vi "Sgl_ErrorCodes&Descs.vi"() -> (0 "Sgl_ErrorsDescs_Trans":T1(array[cluster]) caption="Avantes Error Descriptions (Translated Codes)")   [LabVIEW 2012, in "SG-Lock.lvlib"]
uses:
  SG-Lock.lvlib
panel:
  out "Sgl_ErrorsDescs":T2(array[cluster])=[{"Code"=1, "Name"=enum."SGL_DGL_NOT_FOUND", "Description"="SG-Lock not found"}, {"Code"=2, "Name"=enum."SGL_LPT_BUSY", "Description"="At least one LPT-Port is used by another program and on the other ports no SG-Lock was found"}, {"Code"=3, "Name"=enum."SGL_LPT_OPEN_ERROR", "Description"="The SG-Lock LPT-driver was not found, even though the SGLock LPT support is installed"}, {"Code"=4, "Name"=enum."SGL_NO_LPT_PORT_FOUND", "Description"="There is no LPT-Port installed in the PC, even though the SG-Lock LPT support is installed"}, {"Code"=5, "Name"=enum."SGL_AUTHENTICATION_REQUIRED", "Description"="Authentication with SglAuthent() not or not errorfree processed"}, {"Code"=6, "Name"=enum."SGL_AUTHENTICATION_FAILED", "Description"="Authentication with SglAuthent() failed"}, {"Code"=7, "Name"=enum."SGL_FUNCTION_NOT_SUPPORTED", "Description"="The called function is not supported by the found SG-Lock"}, {"Code"=8, "Name"=enum."SGL_PARAMETER_INVALD", "Description"="Parameter of the called function is out of the vaild value range"}, {"Code"=9, "Name"=enum."SGL_SIGNATURE_INVALID", "Description"="Signature invalid"}, {"Code"=10, "Name"=enum."SGL_USB_BUSY", "Description"="Another application is claming the SG-Lock for more than 5 seconds"}] caption="Avantes Error Descriptions (Directly from Doc)"
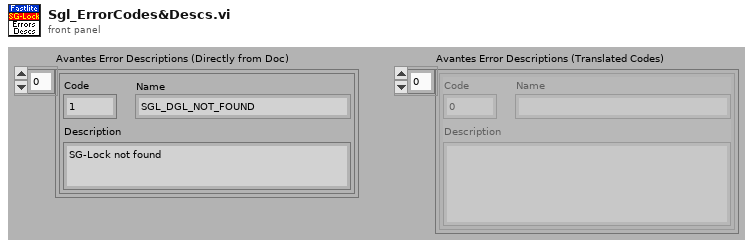
[diagram p1: front panel]
types:
  T1 = cluster{"Code":i32, "Name":string, "Description":string}[]
  T2 = cluster{"Code":i32, "Name":enum16{"SGL_SUCCESS", "SGL_DGL_NOT_FOUND", "SGL_LPT_BUSY", "SGL_LPT_OPEN_ERROR", "SGL_NO_LPT_PORT_FOUND", "SGL_AUTHENTICATION_REQUIRED", "SGL_AUTHENTICATION_FAILED", "SGL_FUNCTION_NOT_SUPPORTED", "SGL_PARAMETER_INVALD", "SGL_SIGNATURE_INVALID", "SGL_USB_BUSY"}, "Description":string}[]
  T3 = cluster{"Code":i32, "Name":string, "Description":string}
  T4 = enum16{"SGL_SUCCESS", "SGL_DGL_NOT_FOUND", "SGL_LPT_BUSY", "SGL_LPT_OPEN_ERROR", "SGL_NO_LPT_PORT_FOUND", "SGL_AUTHENTICATION_REQUIRED", "SGL_AUTHENTICATION_FAILED", "SGL_FUNCTION_NOT_SUPPORTED", "SGL_PARAMETER_INVALD", "SGL_SIGNATURE_INVALID", "SGL_USB_BUSY"}
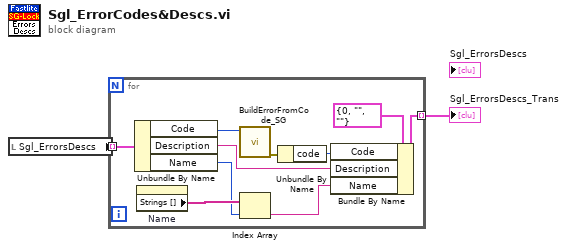
[diagram p0: block diagram]
diagram:
  n1 = local read "Sgl_ErrorsDescs"() -> (w2:T2)
  n2 = for {
    tunnel: w2 -> [w12] mode=indexing
    tunnel: [w10] -> w1 mode=indexing
    n3 = Unbundle By Name(w12) -> ("Code"=w4:i32, "Description"=w7:string, "Name"=w6:T4)
    n4 = property on="Name" class="Enum (strict)"() -> ("Strings []"=w9:string[])  [unwired: 2 in, 2 out]
    n5 = call "BuildErrorFromCode_SG.vi"("Error Code"=w4) -> ("error out"=w3:errorcluster)  [unwired: 10 in]
    n6 = Index Array(array=w9, index=w6) -> (element=w5:string)
    n7 = Unbundle By Name(w3) -> ("code"=w11:i32)
    n8 = Bundle By Name(cluster=T3 {"Code"=0, "Name"="", "Description"=""} ("Cluster"), "Code"=w11, "Description"=w7, "Name"=w5) -> (w10:T3)
  }
  "Sgl_ErrorsDescs_Trans" <- w1
